vi "Get Newest Version.vi"(10 "Version":T1, 11 "Newest Version In":T1) -> (3 "Newest Version Out":T1)   [LabVIEW 2014]
uses:
  <vilib>/AppBuilder/AB_API_Simple/Build Specification Version.ctl
  <vilib>/AppBuilder/AB_API_Simple/NI_App_Builder_API.lvlib
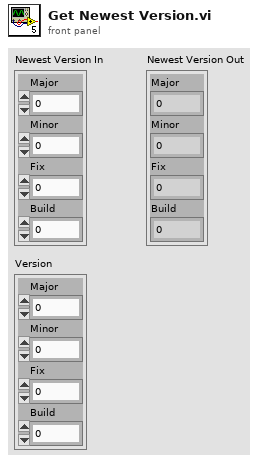
[diagram p1: front panel]
types:
  T1 = typedef "NI_App_Builder_API.lvlib/Build Specification Version.ctl" = cluster{"Major":u16, "Minor":u16, "Fix":u16, "Build":u16}
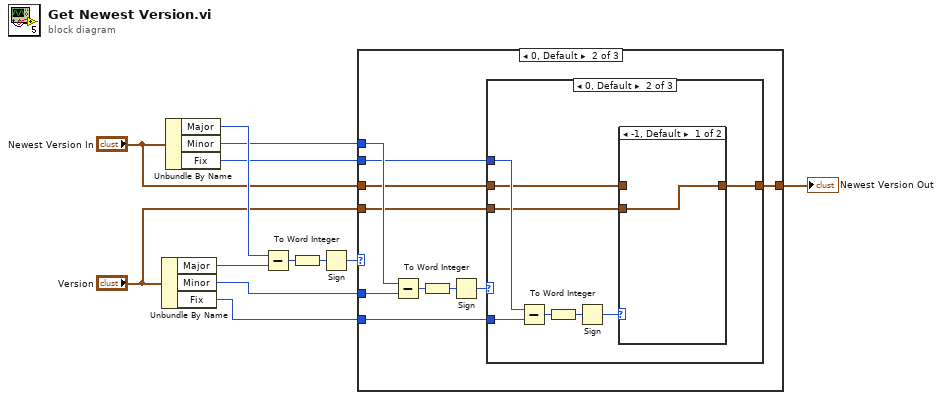
[diagram p0: block diagram]
diagram:
  n1 = Unbundle By Name("Version") -> ("Major"=w12:u16, "Minor"=w7:u16, "Fix"=w6:u16)
  n2 = Unbundle By Name("Newest Version In") -> ("Major"=w11:u16, "Minor"=w9:u16, "Fix"=w8:u16)
  n3 = Subtract(x=w11, y=w12) -> (x-y=w10:u16)
  n4 = To Word Integer(number=w10) -> (16bit integer=w1:i16)
  n5 = Sign(1:w1) -> (0:w5:i16)
  n6 = case shown="0, Default" w5 {
    tunnel: w9 -> [_ w21 _]
    tunnel: w8 -> [_ w15 _]
    tunnel: w7 -> [_ w20 _]
    tunnel: w6 -> [_ w14 _]
    tunnel: "Newest Version In" -> [_ w17 w36]
    tunnel: [w13 w18 w36] -> w3
    tunnel: "Version" -> [w13 w16 _]
    frame -1 {
    }
    frame 0, Default {
      n7 = Subtract(x=w21, y=w20) -> (x-y=w22:u16)
      n8 = To Word Integer(number=w22) -> (16bit integer=w23:i16)
      n9 = Sign(1:w23) -> (0:w19:i16)
      n10 = case shown="0, Default" w19 {
        tunnel: [w24 w27 w35] -> w18
        tunnel: w17 -> [_ w26 w35]
        tunnel: w16 -> [w24 w25 _]
        tunnel: w15 -> [_ w30 _]
        tunnel: w14 -> [_ w29 _]
        frame -1 {
        }
        frame 0, Default {
          n11 = Subtract(x=w30, y=w29) -> (x-y=w32:u16)
          n12 = To Word Integer(number=w32) -> (16bit integer=w31:i16)
          n13 = Sign(1:w31) -> (0:w28:i16)
          n14 = case shown="-1, Default" w28 {
            tunnel: [w33 w34] -> w27
            tunnel: w26 -> [_ w34]
            tunnel: w25 -> [w33 _]
            frame -1, Default {
            }
            frame 0, 1 {
            }
          }
        }
        frame 1 {
        }
      }
    }
    frame 1 {
    }
  }
  "Newest Version Out" <- w3
